vi "Acquire Data from Hardware.vi"(10 "User Specified":T1={"Hardware Configuration"={"Signal Channel"="PXI1Slot7/ao0", "Response Channel"="PXI1Slot7/ai0", "Trigger Channel"="/PXI1Slot7/PFI0", "Number of Acquisitions"=0.0}, "Analysis Configuration"={"Statistics"=TRUE}, "Signal Type"=enum."Single Chirp", "New Data Behavior"=enum."Replace", "Signal Configuration"={"Chirp Amplitude"=0.1, "I/O Limit"=10.0, "Sample Rate"=1000000.0, "Chirp Duration (s)"=10000000.0, "Upper Frequency"=0.0, "Lower Frequency"=0.0, "Windowing"=enum."None"}}) -> (0 "error out":errorcluster, 2 "Waveform Graph":dynamicdata(graph))   [LabVIEW 2017]
doc: "Generates sample waveforms according to the signal type in the HW Config input."
uses:
  controls/User Specified Data.ctl
  controls/HW Configuration.ctl
  controls/Analysis Configuration.ctl
  controls/New Data Behavior.ctl
  controls/Signal Configuration.ctl
  <vilib>/DAQmx/write.llb/DAQmx Write (Analog Wfm 1Chan NSamp).vi
  <vilib>/DAQmx/read.llb/DAQmx Read (Analog Wfm 1Chan NSamp).vi
  <vilib>/DAQmx/create/channels.llb/DAQmx Create Channel (AO-Voltage-Basic).vi
  <vilib>/DAQmx/configure/timing.llb/DAQmx Timing (Sample Clock).vi
  <vilib>/DAQmx/miscellaneous.llb/DAQmx Fill In Error Info.vi
  <vilib>/DAQmx/configure/trigger.llb/DAQmx Start Trigger (Digital Edge).vi
  <vilib>/DAQmx/create/channels.llb/DAQmx Create Channel (AI-Voltage-Basic).vi
panel:
  in  "error in":errorcluster
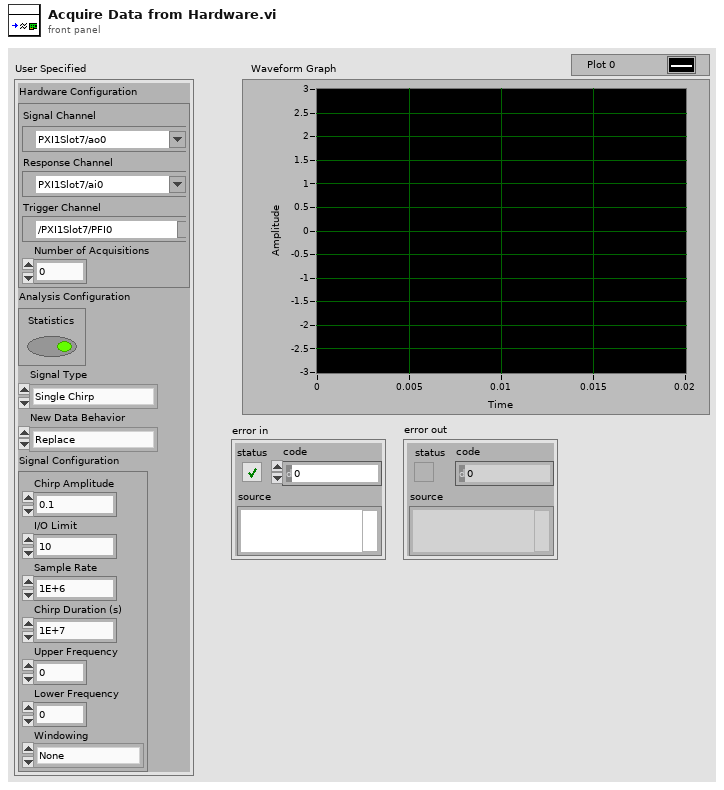
[diagram p1: front panel]
types:
  T1 = typedef "User Specified Data.ctl" = cluster{"Hardware Configuration":T2, "Analysis Configuration":T3, "Signal Type":enum16{"Single Chirp", "From Excel"}, "New Data Behavior":T4, "Signal Configuration":T5}
  T2 = typedef "HW Configuration.ctl" = cluster{"Signal Channel":tag, "Response Channel":tag, "Trigger Channel":tag, "Number of Acquisitions":dbl}
  T3 = typedef "Analysis Configuration.ctl" = cluster{"Statistics":bool}
  T4 = typedef "New Data Behavior.ctl" = enum16{"Replace", "Overlay", "Append"}
  T5 = typedef "Signal Configuration.ctl" = cluster{"Chirp Amplitude":dbl, "I/O Limit":dbl, "Sample Rate":dbl, "Chirp Duration (s)":dbl, "Upper Frequency":dbl, "Lower Frequency":dbl, "Windowing":enum16{"None", "Exponential", "Flat top", "Hamming", "Hanning", "Kaiser-Bessel", "Rectangular"}}
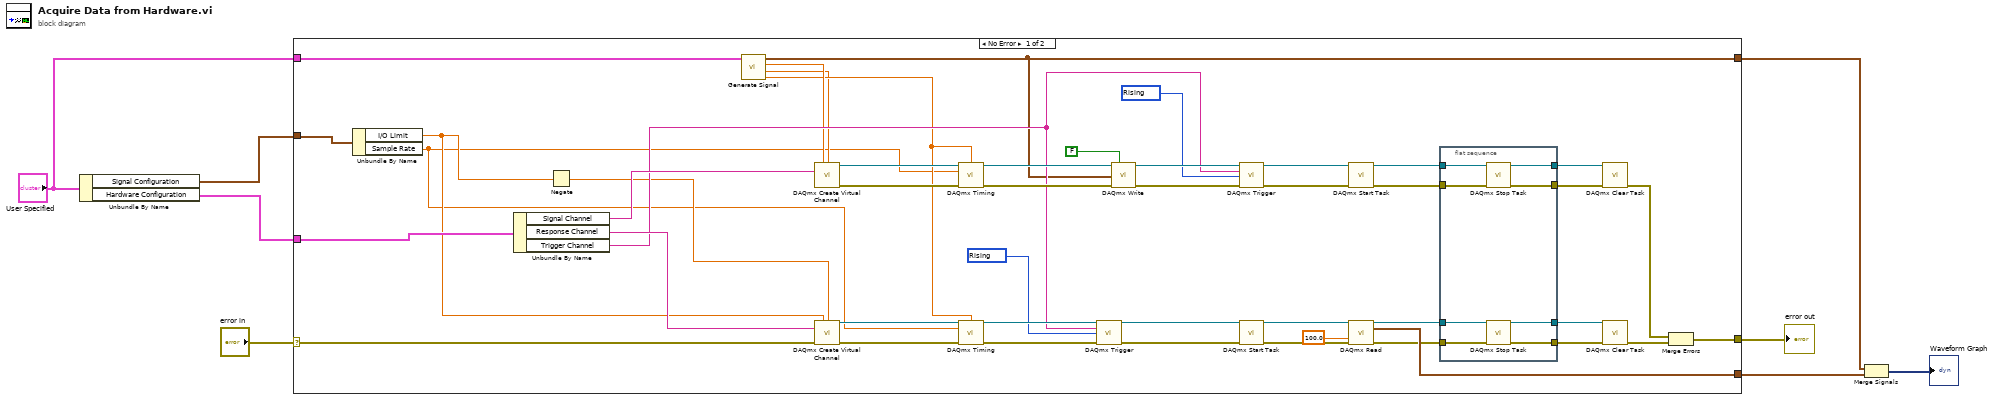
[diagram p0: block diagram]
diagram:
  n1 = Unbundle By Name("User Specified") -> ("Signal Configuration"=w3:T5, "Hardware Configuration"=w2:T2)
  n2 = case shown="No Error" "error in" {
    selector: "error in" -> [w51 w63]
    tunnel: w2 -> [w54 _]
    tunnel: [w43 w63] -> w8
    tunnel: [w32 _] -> w6
    tunnel: [w17 _] -> w4
    tunnel: w3 -> [w16 _]
    tunnel: "User Specified" -> [w14 _]
    frame No Error {
      w21 = 10280 items=["Rising"=10280, "Falling"=10171] ("edge")
      w22 = 10280 items=["Rising"=10280, "Falling"=10171] ("edge")
      n3 = Unbundle By Name(w16) -> ("I/O Limit"=w15:dbl, "Sample Rate"=w10:dbl)
      n4 = Unbundle By Name(w54) -> ("Signal Channel"=w47:tag, "Response Channel"=w50:tag, "Trigger Channel"=w20:tag)
      n5 = Negate(x=w15) -> (-x=w18:dbl)
      n6 = call "Generate Signal.vi"("User Specified"=w14) -> ("Number of samples"=w12:dbl, "Y min"=w11:dbl, "Y max"=w13:dbl, "Final Waveform"=w17:waveform(dbl))  [unwired: 7 in]
      n7 = call-poly <vilib>:"DAQmx Create Virtual Channel.vi"("maximum value"=w13, "minimum value"=w11, "physical channels"=w47) -> ("task out"=w46:refnum<k21>, "error out"=w45:errorcluster)  [unwired: 11 in]
      n8 = call-poly <vilib>:"DAQmx Create Virtual Channel.vi"("maximum value"=w15, "minimum value"=w18, "physical channels"=w50, "error in"=w51) -> ("task out"=w48:refnum<k21>, "error out"=w49:errorcluster)  [unwired: 10 in]
      n9 = call-poly <vilib>:"DAQmx Timing.vi"("task/channels in"=w46, "samples per channel"=w12, "rate"=w10, "error in"=w45) -> ("task out"=w42:refnum<k21>, "error out"=w41:errorcluster)  [unwired: 10 in]
      n10 = call-poly <vilib>:"DAQmx Timing.vi"("task/channels in"=w48, "samples per channel"=w12, "rate"=w10, "error in"=w49) -> ("task out"=w30:refnum<k21>, "error out"=w29:errorcluster)  [unwired: 10 in]
      n11 = call-poly <vilib>:"DAQmx Trigger.vi"("task/channels in"=w30, "source"=w20, "edge"=w21, "error in"=w29) -> ("task out"=w27:refnum<k21>, "error out"=w28:errorcluster)  [unwired: 10 in]
      n12 = call-poly <vilib>:"DAQmx Write.vi"("task/channels in"=w42, "auto start"=FALSE, "data"=w17, "error in"=w41) -> ("task out"=w26:refnum<k21>, "error out"=w25:errorcluster)  [unwired: 9 in, 1 out]
      n13 = call-poly <vilib>:"DAQmx Trigger.vi"("task/channels in"=w26, "source"=w20, "edge"=w22, "error in"=w25) -> ("task out"=w23:refnum<k21>, "error out"=w24:errorcluster)  [unwired: 10 in]
      n14 = call <vilib>:"DAQmx Start Task.vi"("task/channels in"=w27, "error in"=w28) -> ("task out"=w35:refnum<k21>, "error out"=w34:errorcluster)  [unwired: 12 in]
      n15 = call <vilib>:"DAQmx Start Task.vi"("task/channels in"=w23, "error in"=w24) -> ("task out"=w37:refnum<k21>, "error out"=w36:errorcluster)  [unwired: 12 in]
      n16 = call-poly <vilib>:"DAQmx Read.vi"("task/channels in"=w35, "timeout"=100.0, "error in"=w34) -> ("task out"=w33:refnum<k21>, "data"=w32:waveform(dbl), "error out"=w31:errorcluster)  [unwired: 10 in]
      n17 = flat-sequence {
        tunnel: [w62] -> w53
        tunnel: [w61] -> w52
        tunnel: [w60] -> w40
        tunnel: [w59] -> w38
        tunnel: w37 -> [w58]
        tunnel: w36 -> [w57]
        tunnel: w33 -> [w56]
        tunnel: w31 -> [w55]
        frame #0 {
          n18 = call <vilib>:"DAQmx Stop Task.vi"("task/channels in"=w58, "error in"=w57) -> ("task out"=w59:refnum<k21>, "error out"=w60:errorcluster)  [unwired: 12 in]
          n19 = call <vilib>:"DAQmx Stop Task.vi"("task/channels in"=w56, "error in"=w55) -> ("task out"=w61:refnum<k21>, "error out"=w62:errorcluster)  [unwired: 12 in]
        }
      }
      n20 = call <vilib>:"DAQmx Clear Task.vi"("task in"=w38, "error in"=w40) -> ("error out"=w39:errorcluster)  [unwired: 13 in]
      n21 = call <vilib>:"DAQmx Clear Task.vi"("task in"=w52, "error in"=w53) -> ("error out"=w44:errorcluster)  [unwired: 13 in]
      n22 = Merge Errors(w39, w44) -> (w43:errorcluster)
    }
    frame Error {
    }
  }
  "error out" <- w8
  n23 = Merge Signals(w4, w6) -> (→"Waveform Graph":dynamicdata)
